vi "SetInputChannels.vi"(7 "Channels":T1[](array[typedef]) {"DeadTime" min=800 max=160000 step=1; "Edge" items=["falling", "rising"]; "Offset" min=-100000 max=100000 step=10; "Level" min=-1200 max=1200 step=1}, 8 "error in (no error)":errorcluster, 9 "SetInpChan":T2[](array[typedef]), 10 "features":i32, 11 "Multiharp in":refnum<class "Multiharp.lvclass">) -> (0 "error out":errorcluster, 3 "Multiharp out":refnum<class "Multiharp.lvclass">)   [LabVIEW 2023, in "Multiharp.lvlib" / "Multiharp.lvclass"]
uses:
  Multiharp.lvclass
  <vilib>/ActorFramework/Actor/Actor.lvclass
  Multiharp Messages/SetSyncDivider Msg/SetSyncDivider Msg.lvclass
  Types/MH_SetInpChanCmds.ctl
  Types/MH_SetInpChanData.ctl
  Types/MH_InputChannel.ctl
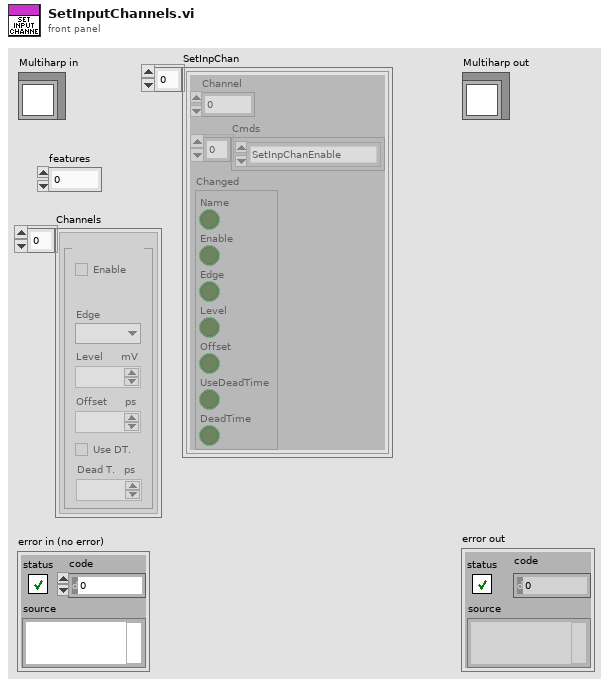
[diagram p1: front panel]
types:
  T1 = typedef "MH_InputChannel.ctl" = cluster{"Name":string, "Enable":bool, "Edge":i32, "Level":i32, "Offset":i32, "UseDeadTime":bool, "DeadTime":i32}
  T2 = typedef "MH_SetInpChanData.ctl" = cluster{"Channel":i32, "Cmds":T3[], "Changed":cluster{"Name":bool, "Enable":bool, "Edge":bool, "Level":bool, "Offset":bool, "UseDeadTime":bool, "DeadTime":bool}}
  T3 = typedef "MH_SetInpChanCmds.ctl" = enum16{"SetInpChanEnable", "SetInpChanOffset", "SetInpChanDeadTime", "SetInpChanTrg"}
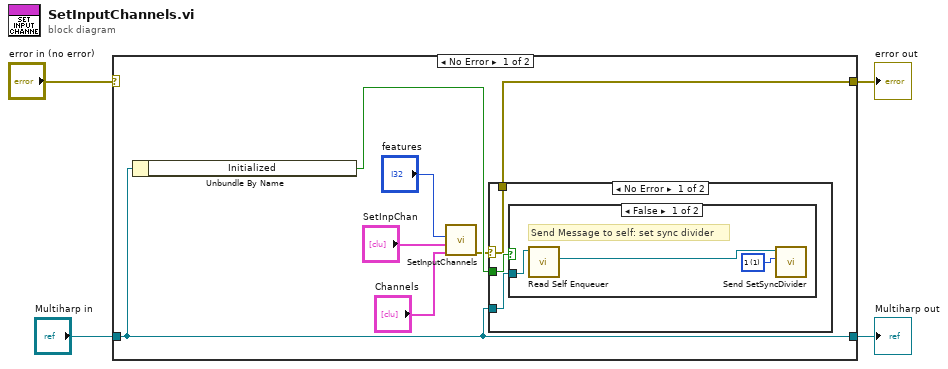
[diagram p0: block diagram]
diagram:
  n1 = case shown="No Error" "error in (no error)" {
    selector: "error in (no error)" -> [_ w20]
    tunnel: [w5 w20] -> w3
    tunnel: [w11 w19] -> w1
    tunnel: "Multiharp in" -> [w11 w19]
    frame No Error {
      n2 = Unbundle By Name(w11) -> ("Initialized"=w10:bool)
      n3 = call "SetInputChannels.vi"("Channels"="Channels", "SetInpChan"="SetInpChan", "features"="features") -> ("error out"=w6:errorcluster)  [unwired: 8 in]
      n4 = case shown="No Error" w6 {
        selector: w6 -> [w12 w18]
        tunnel: w11 -> [w14 _]
        tunnel: w10 -> [w13 _]
        tunnel: [w12 w18] -> w5
        frame No Error {
          n5 = case shown="False" w13 {
            tunnel: w14 -> [w17 _]
            frame False {
              w15 = 1 items=["1"=1, "2"=2, "4"=4, "8"=8, "16"=16] ("SyncDivider")
              # "Send Message to self: set sync divider"
              n6 = call <vilib>:"Read Self Enqueuer.vi"("Actor"=w17) -> ("Self Enqueuer"=w16:refnum<class "Message Enqueuer.lvclass">)  [unwired: 10 in]
              n7 = call "Send SetSyncDivider.vi"("SyncDivider"=w15, "Message Enqueuer"=w16) -> ()  [unwired: 8 in, 2 out]
            }
            frame True {
              # "Send message to Controller"
            }
          }
        }
        frame Error {
        }
      }
    }
    frame Error {
    }
  }
  "error out" <- w3
  "Multiharp out" <- w1
